vi "SL_WriteData.vi"(9 "Data":string caption="Data In", 10 "Type":string, 11 "Path":string) -> ()   [LabVIEW 2020]
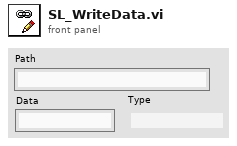
[diagram p1: front panel]
types:
  T1 = cluster{"timestamp":string, "value":cluster{"type":string, "value":string}}
  T2 = enum16{"GET", "PUT", "POST", "MultiPOST", "DELETE"}
  T3 = cluster{"Name":string, "BaseURL":string, "AppKey":string, "Headers":string[], "Timeout":i32}
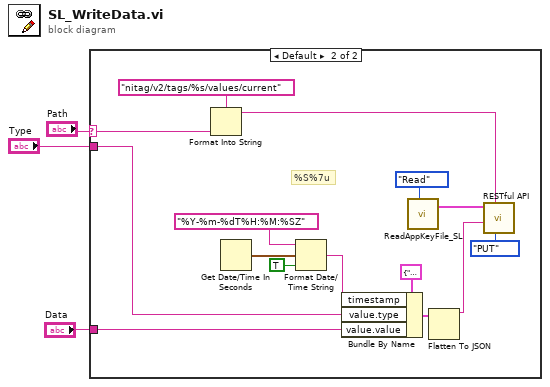
[diagram p0: block diagram]
diagram:
  n1 = case shown="Default" "Path" {
    selector: "Path" -> [_ w8]
    tunnel: "Type" -> [_ w6]
    tunnel: "Data" -> [_ w4]
    frame "" {
    }
    frame Default {
      # "%S%7u"
      n2 = Format Into String(format string="nitag/v2/tags/%s/values/current" ("url"), w8) -> (resulting string=w7:string)  [unwired: 2 in, 1 out]
      n3 = Get Date/Time In Seconds() -> (seconds since 1Jan1904=w13:timestamp)
      n4 = Format Date/Time String(time format string (%c)="%Y-%m-%dT%H:%M:%SZ", seconds (now)=w13, UTC format=TRUE) -> (date/time string=w15:string)
      n5 = Bundle By Name(cluster=T1 {"timestamp"="", "value"={"type"="", "value"=""}}, "timestamp"=w15, "value.type"=w6, "value.value"=w4) -> (w11:T1)
      n6 = call "ReadAppKeyFile_SL.vi"("Task"=enum16{"Read", "Write"}."Read") -> ("Device Out"=w5:T3)  [unwired: 8 in, 2 out]
      n7 = Flatten To JSON(anything=w11) -> (JSON string=w9:string)  [unwired: 2 in, 1 out]
      n8 = call "RESTful API.vi"("Method"=T2."PUT", "url"=w7, "JSON"=w9, "Device In"=w5) -> ()  [unwired: 5 in, 3 out]
    }
  }
